vi "steps.vi"(0 "COM Bluegiga in":refnum<visa-resource-name>, 5 "error in (no error)":errorcluster) -> (14 "COM Bluegiga out":refnum<visa-resource-name>, 16 "Tiempo":u32, 17 "Pasos":u32, 19 "error out":errorcluster)   [LabVIEW 2020]
panel:
  out "characteristic value":u8[](array[numeric])
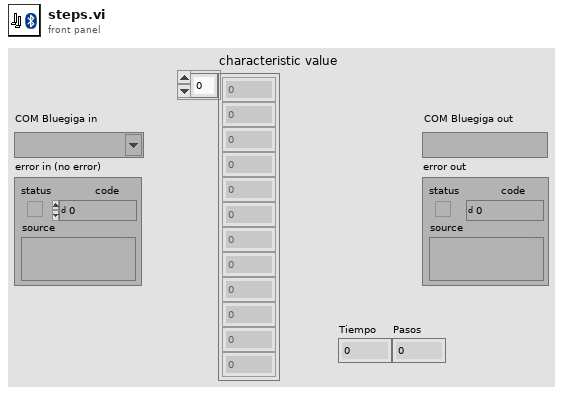
[diagram p1: front panel]
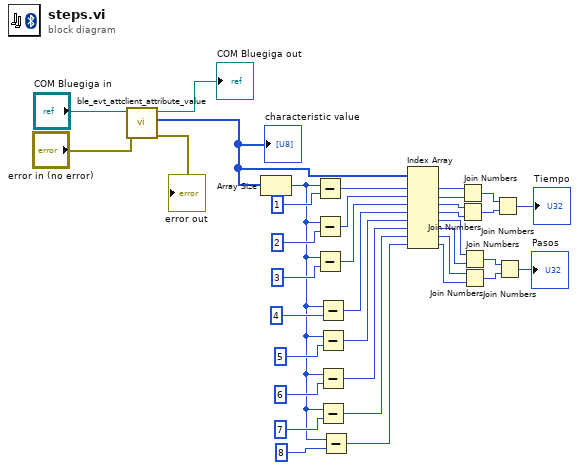
[diagram p0: block diagram]
diagram:
  n1 = call <vilib>:"ble_evt_attclient_attribute_value.vi"("error in (no error)"="error in (no error)", "COM Bluegiga in"="COM Bluegiga in") -> ("error out"=→"error out":errorcluster, "characteristic value"=w34:u8[], "COM Bluegiga out"=→"COM Bluegiga out":refnum<visa-resource-name>)  [unwired: 6 in, 1 out]
  "characteristic value" <- w34
  n2 = Array Size(array=w34) -> (size(s)=w5:i32)
  n3 = Subtract(x=w5, y=1) -> (x-y=w36:i32)
  n4 = Subtract(x=w5, y=2) -> (x-y=w26:i32)
  n5 = Subtract(x=w5, y=3) -> (x-y=w25:i32)
  n6 = Subtract(x=w5, y=4) -> (x-y=w24:i32)
  n7 = Subtract(x=w5, y=5) -> (x-y=w4:i32)
  n8 = Subtract(x=w5, y=6) -> (x-y=w3:i32)
  n9 = Subtract(x=w5, y=7) -> (x-y=w2:i32)
  n10 = Subtract(x=w5, y=8) -> (x-y=w1:i32)
  n11 = Index Array(array=w34, index #1=w36, index #2=w26, index #3=w25, index #4=w24, index #5=w4, index #6=w3, index #7=w2, index #8=w1) -> (element #1=w20:u8, element #2=w21:u8, element #3=w22:u8, element #4=w23:u8, element #5=w13:u8, element #6=w12:u8, element #7=w11:u8, element #8=w10:u8)
  n12 = Join Numbers(hi=w20, lo=w21) -> ((hi.lo)=w18:u16)
  n13 = Join Numbers(hi=w22, lo=w23) -> ((hi.lo)=w19:u16)
  n14 = Join Numbers(hi=w13, lo=w12) -> ((hi.lo)=w15:u16)
  n15 = Join Numbers(hi=w11, lo=w10) -> ((hi.lo)=w16:u16)
  n16 = Join Numbers(hi=w18, lo=w19) -> ((hi.lo)=→"Tiempo":u32)
  n17 = Join Numbers(hi=w15, lo=w16) -> ((hi.lo)=→"Pasos":u32)
